vi "3A PWM MotorControl FPGA.vi"() -> ()   [LabVIEW 2011]
uses:
  <vilib>/robotics/Utilities/FPGA Utilities/Generate Digital Pulse (uSec).vi
  <vilib>/robotics/Utilities/FPGA Utilities/NI_Robotics_FPGA Utilities.lvlib
panel:
  in  "SERVO 2 Duty in Ticks":u32
  in  "stop PWM":bool
  in  "SERVO 1 Duty in Ticks":u32
  # "Winch"
  # "Rudder"
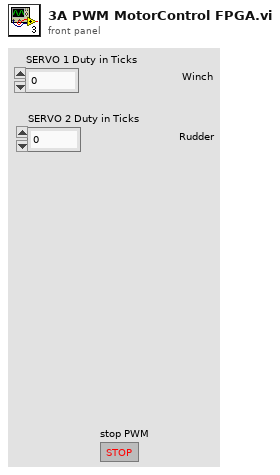
[diagram p1: front panel]
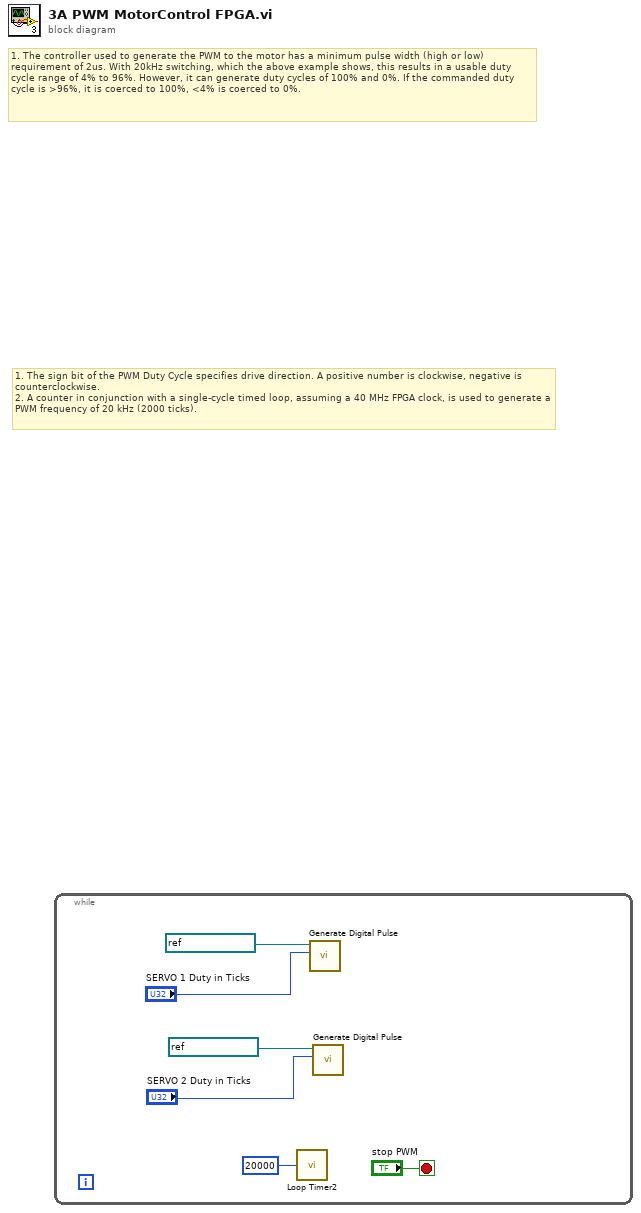
[diagram p0: block diagram]
diagram:
  # "1. The sign bit of the PWM Duty Cycle specifies drive direction. A positive number is clockwise, negative is counterclockwise.\n2. A counter in conjunction with a single-cycle timed loop, assuming a 40 MHz FPGA clock, is used to generate a PWM frequency of 20 kHz (2000 ticks)."
  # "1. The controller used to generate the PWM to the motor has a minimum pulse width (high or low) requirement of 2us. With 20kHz switching, which the above example shows, this results in a usable duty cycle range of 4% to 96%. However, it can generate duty cycles of 100% and 0%. If the commanded duty cycle is >96%, it is coerced to 100%, <4% is coerced to 0%."
  n1 = while {
    stop <- "stop PWM" stop-if-true
    n2 = call "Loop Timer2"("Count(uSec)"=u32 20000) -> ()  [unwired: 1 out]
    n3 = call-poly <vilib>:"Generate Digital Pulse.vi"("pulse width (uSec)"="SERVO 1 Duty in Ticks", "FPGA digital output"=refnum<k21> "Mod4/DIO0") -> ()  [unwired: 10 in]
    n4 = call-poly <vilib>:"Generate Digital Pulse.vi"("pulse width (uSec)"="SERVO 2 Duty in Ticks", "FPGA digital output"=refnum<k21> "Mod4/DIO1") -> ()  [unwired: 10 in]
  }
